vi "SimpleConnectAndSubscribe.vi"() -> ()   [LabVIEW 2018, in "AWS_IoT.lvlib"]
doc: "A basic client example that connects to a server, subscribes to a variety of topics and receives responses for the topics. \n\n© 2015 - daq.io, LLC - Peter Adelhardt"
uses:
  AWS_IoT.lvlib
  MQTT/Controls/QoS.ctl
  MQTT/Controls/MessageType.ctl
  MQTT/Controls/Connection_Return_Codes.ctl
  Controls/certs.ctl
  MQTT/Controls/ConnectMeta.ctl
  MQTT/Controls/Retain_Flag.ctl
  MQTT/Controls/DUP_Flag.ctl
  MQTT/Controls/Connect_Flags.ctl
panel:
  out "msg ct":i32
  in  "cert path":T1={"client cert file"=path "", "client key file"=path ""}
  out "Connection Status":T2=enum."Connection refused: not authorized"
  out "Messages":T4(array[cluster])
  in  "Stop Reading":bool
  in  "MQTT Broker":cluster{"address (IP)":string, "port":u16}={"address (IP)"="a28e3t2sj3ekjh.iot.us-west-2.amazonaws.com", "port"=8883}
  in  "Subscription Info Array":cluster{"Topic":string, "QoS":T5}[](array[cluster])=[{"Topic"="testtopic/LVMQTT", "QoS"=enum."At most once"}]
  out "Granted QoS Levels":T5[](array[typedef])
  in  "Client ID":string="LVSubscribeClient"
  out "error out":errorcluster
  in  "error in (no error)":errorcluster
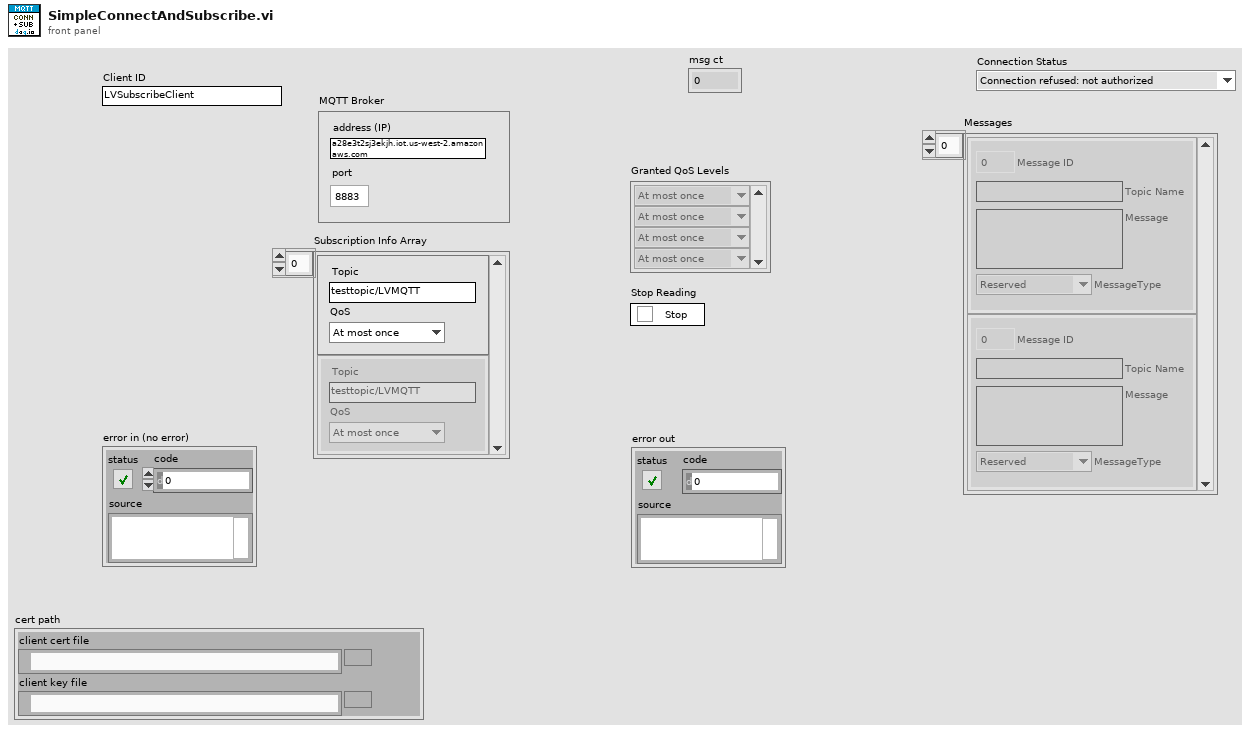
[diagram p1: front panel]
types:
  T1 = typedef "AWS_IoT.lvlib/certs.ctl" = cluster{"client cert file":path, "client key file":path}
  T2 = typedef "AWS_IoT.lvlib/Connection_Return_Codes.ctl" = enum16{"Connection accepted", "Connection refused: unacceptable protocol version", "Connection refused: identifier rejected", "Connection refused: Server unavailable", "Connection refused: bad user name or password", "Connection refused: not authorized"}
  T3 = typedef "AWS_IoT.lvlib/MessageType.ctl" = enum32{"Reserved", "CONNECT", "CONNACK", "PUBLISH", "PUBACK", "PUBREC", "PUBREL", "PUBCOMP", "SUBSCRIBE", "SUBACK", "UNSUBSCRIBE", "UNSUBACK", "PINGREQ", "PINGRESP", "DISCONNECT", "Reserved2"}
  T4 = cluster{"Message ID":u16, "Topic Name":string, "Message ":string, "MessageType":T3}[]
  T5 = typedef "AWS_IoT.lvlib/QoS.ctl" = enum8{"At most once", "At least once", "Exactly once", "Reserved"}
  T6 = cluster{"Message ID":u16, "Topic Name":string, "Message":string, "MessageType":T3}
  T7 = typedef "AWS_IoT.lvlib/Connect_Flags.ctl" = cluster{"user name":bool, "password":bool, "will retain":bool, "will flag":bool, "clean session":bool, "reserved":bool, "will QoS":T5}
  T8 = typedef "AWS_IoT.lvlib/ConnectMeta.ctl" = cluster{"Retain":T9, "DUP":T10, "Keep Alive (sec)":u16, "QoS":T5}
  T9 = typedef "AWS_IoT.lvlib/Retain_Flag.ctl" = bool
  T10 = typedef "AWS_IoT.lvlib/DUP_Flag.ctl" = bool
  T11 = typedef "AWS_IoT.lvlib/SSL_Connection.ctl" = cluster{"connection ID":refnum<k5>, "TLS":cluster{"CXT ptr":i32, "SSL ptr":i32, "Socket ptr":i32}, "NIssleay library path":path, "server url":string}
  T12 = cluster{"Message ID":u16, "Topic Name":string, "Message":string, "MessageType":T3}[]
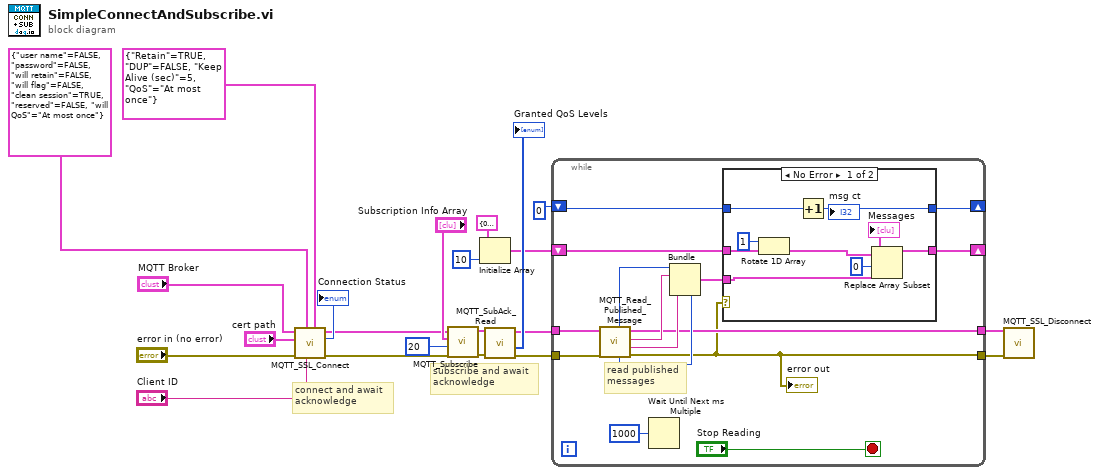
[diagram p0: block diagram]
diagram:
  # "connect and await\nacknowledge"
  # "subscribe and await\nacknowledge"
  n1 = call "MQTT_SSL_Connect.vi"("Connect Meta"=T8 {"Retain"=TRUE, "DUP"=FALSE, "Keep Alive (sec)"=5, "QoS"=enum."At most once"}, "Client ID"="Client ID", "Connect Flags"=T7 {"user name"=FALSE, "password"=FALSE, "will retain"=FALSE, "will flag"=FALSE, "clean session"=TRUE, "reserved"=FALSE, "will QoS"=enum."At most once"}, "error in (no error)"="error in (no error)", "cert path"="cert path", "MQTT Broker"="MQTT Broker") -> ("error out"=w11:errorcluster, "Connection Status"=→"Connection Status":T2, "SSL_Connection"=w10:T11)  [unwired: 3 in]
  n2 = call "MQTT_Subscribe.vi"("error in (no error)"=w11, "Message ID"=u16 20, "Subscription Info Array"="Subscription Info Array", "SSL_Connection"=w10) -> ("error out"=w14:errorcluster, "SSL_Connection"=w9:T11)  [unwired: 6 in]
  n3 = Initialize Array(T6 {"Message ID"=0, "Topic Name"="", "Message"="", "MessageType"=enum."Reserved"}, 10 ("dimension size")) -> (w2:T12)
  n4 = call "MQTT_SubAck_Read.vi"("error in (no error)"=w14, "SSL_Connection"=w9) -> ("error out"=w19:errorcluster, "Granted QoS Levels"=→"Granted QoS Levels":T5[], "SSL_Connection 2"=w18:T11)  [unwired: 7 in]
  n5 = while {
    shift-right: [w34] -> _
    shift-left: w2 -> [w36]
    tunnel: w19 -> [w32]
    tunnel: [w25] -> w17
    tunnel: w18 -> [w33]
    tunnel: [w27] -> w8
    shift-right: [w23] -> _
    shift-left: 0 -> [w24]
    stop <- "Stop Reading" stop-if-true
    # "read published\nmessages"
    n6 = call "MQTT_Read_Published_Message.vi"("error in (no error)"=w32, "SSL_Connection"=w33) -> ("error out"=w25:errorcluster, "Message"=w31:string, "Topic Name"=w30:string, "SSL_Connection"=w27:T11, "MessageType"=w28:T3, "Message ID"=w29:u16)  [unwired: 4 in]
    "error out" <- w25
    n7 = Wait Until Next ms Multiple(millisecond multiple=u32 1000) -> ()  [unwired: 1 out]
    n8 = Bundle("Message ID"=w29, "Topic Name"=w30, "Message"=w31, "MessageType"=w28) -> (w35:T6)  [unwired: 1 in]
    n9 = case shown="No Error" w25 {
      tunnel: w36 -> [w45 w47]
      tunnel: w35 -> [w43 _]
      tunnel: [w44 w47] -> w34
      tunnel: w24 -> [w39 w46]
      tunnel: [w38 w46] -> w23
      frame No Error {
        n10 = Rotate 1D Array(1:w45, 2:1 ("n")) -> (0:w41:T12)
        n11 = Increment(x=w39) -> (x+1=w38:i32)
        "msg ct" <- w38
        n12 = Replace Array Subset(array=w41, new element=w43, index=0) -> (w44:T12)
        "Messages" <- w44
      }
      frame Error {
      }
    }
  }
  n13 = call "MQTT_SSL_Disconnect.vi"("error in (no error)"=w17, "SSL_Connection"=w8) -> ()  [unwired: 9 in, 1 out]
